vi "glb_ClientSrv Globals.vi"() -> ()   [LabVIEW 2012]
panel:
  in  "client info":string
  out "reboot":bool
  in  "client VI ref":refnum<vi>
  in  "client version":string
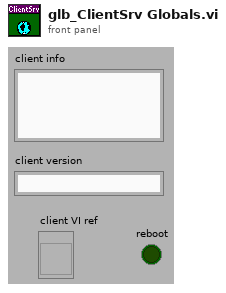
[diagram p1: front panel]
diagram:
